vi "XNET Convert (Signal to Frame LIN).vi"(0 "session in":refnum<k21>, 5 "signal data":dbl[](array[numeric]) format="%.2f", 11 "error in (no error)":errorcluster) -> (4 "session out":refnum<k21>, 6 "frame data":T1[](array[typedef]) {"event ID" format="%x"; "payload" format="%x"; "timestamp" format="%<%.7X\n%x>T"; "type" items=["LIN Data"=64, "LIN Bus Error"=65, "LIN No Response"=66, "Delay"=224, "Log Trigger"=225, "Start Trigger"=226]; "identifier" format="%x"}, 14 "unused payloads":cluster{"payload":u8[]}[](array[cluster]), 15 "error out":errorcluster)   [LabVIEW 2018]
doc: "Converts signal data to NI-XNET LIN frame data."
uses:
  XNET Frame LIN.ctl
  XNET Frame Type LIN.ctl
  nixlvapi.dll
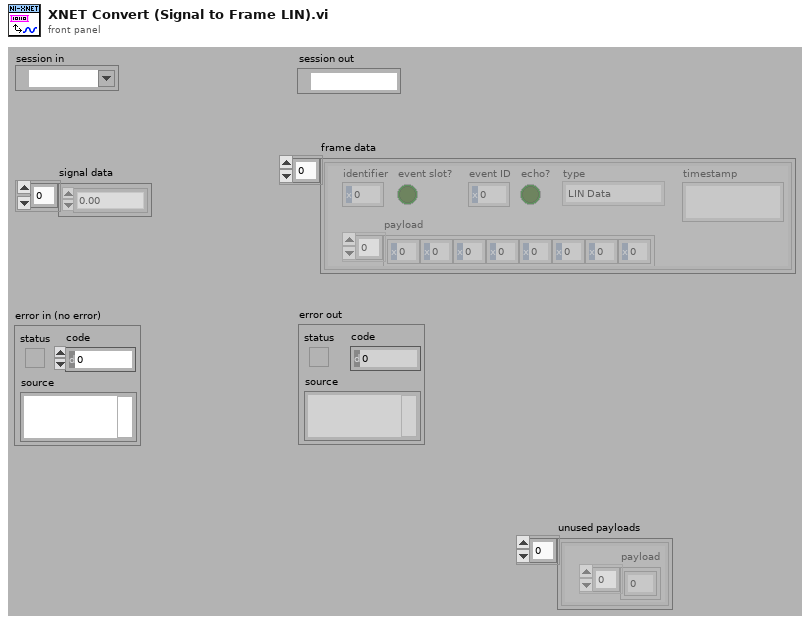
[diagram p1: front panel]
types:
  T1 = typedef "XNET Frame LIN.ctl" = cluster{"timestamp":timestamp, "payload":u8[], "identifier":u32, "type":T2, "event ID":u8, "event slot?":bool, "echo?":bool}
  T2 = typedef "XNET Frame Type LIN.ctl" = u8
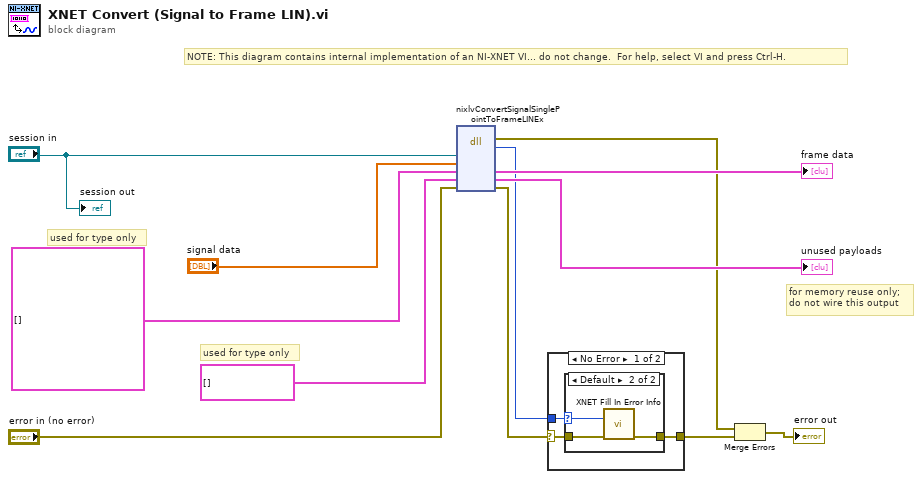
[diagram p0: block diagram]
diagram:
  # "used for type only"
  # "for memory reuse only;\ndo not wire this output"
  # "used for type only"
  # "NOTE: This diagram contains internal implementation of an NI-XNET VI... do not change.  For help, select VI and press Ctrl-H."
  n1 = dll-call lib="nixlvapi.*" fn="nixlvConvertSignalSinglePointToFrameLINEx" label="Call Library"("sessionRef"="session in", "signalData"="signal data", "frameData"=T1[] [] ("data"), "unusedPayloads"=cluster{"payload":u8[]}[] [] ("payload array"), "errorInOut"="error in (no error)") -> (error out=w1:errorcluster, "return type"=w4:i32, "frameData"=→"frame data":T1[], "unusedPayloads"=→"unused payloads":cluster{"payload":u8[]}[], "errorInOut"=w3:errorcluster)  [unwired: 4 in, 2 out]
  n2 = case shown="No Error" w3 {
    selector: w3 -> [w13 w20]
    tunnel: [w15 w20] -> w12
    tunnel: w4 -> [w14 _]
    frame No Error {
      n3 = case shown="Default" w14 {
        selector: w14 -> [_ w17]
        tunnel: w13 -> [w16 w18]
        tunnel: [w16 w19] -> w15
        frame 0 {
        }
        frame Default {
          n4 = call "XNET Fill In Error Info.vi"("status code"=w17, "error in"=w18) -> ("error out"=w19:errorcluster)  [unwired: 13 out]
        }
      }
    }
    frame Error {
    }
  }
  n5 = Merge Errors(w1, w12) -> (→"error out":errorcluster)
  "session out" <- "session in"
